vi "DB2Sin.vi"(10 "amplitude":dbl=1.0 format="%#_13g", 11 "DB Data":dbl[][](array[numeric])) -> (3 "sine wave":dbl[](array[numeric]))   [LabVIEW 2020]
uses:
  <vilib>/measure/NI_MABase.lvlib
panel:
  out "Waveform Graph":waveform(dbl)(graph)
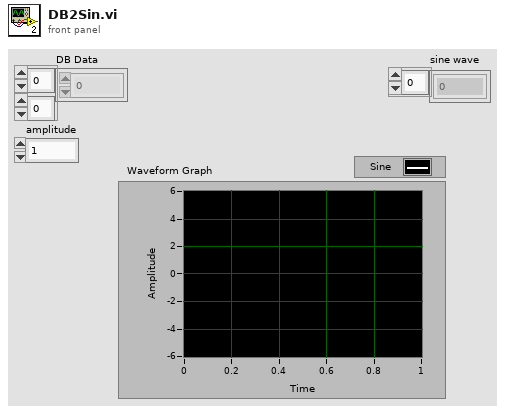
[diagram p1: front panel]
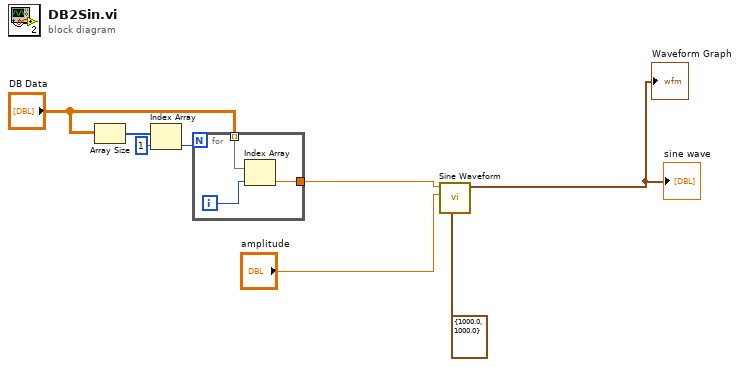
[diagram p0: block diagram]
diagram:
  n1 = Array Size(array="DB Data") -> (size(s)=w7:i32[])
  n2 = Index Array(array=w7, index=1) -> (element=w8:i32)
  n3 = for {
    N: w8 -> [_]
    tunnel: "DB Data" -> [w10] mode=indexing
    tunnel: [w9] -> w3
    i -> [w11]
    n4 = Index Array(array=w10, index=w11) -> (element=w9:dbl)
  }
  n5 = call <vilib>:"Sine Waveform.vi"("sampling info"=cluster{"Fs":dbl, "#s":dbl} {"Fs"=1000.0, "#s"=1000.0}, "amplitude"="amplitude", "frequency"=w3) -> ("signal out"=→"sine wave" →"Waveform Graph":waveform(dbl))  [unwired: 7 in, 1 out]
